vi "InitDC.vi"(8 "error in (no error)":errorcluster, 9 "_addr":u8, 10 "Motornum":u8, 11 "DCMotor in":refnum<class "DCMotor.lvclass">) -> (0 "error out":errorcluster, 3 "DCMotor out":refnum<class "DCMotor.lvclass">)   [LabVIEW 2022 SP3, in "Motorshield.lvlib" / "DCMotor.lvclass"]
uses:
  DCMotor.lvclass
  DCMotor.lvclass/DCMotor.ctl
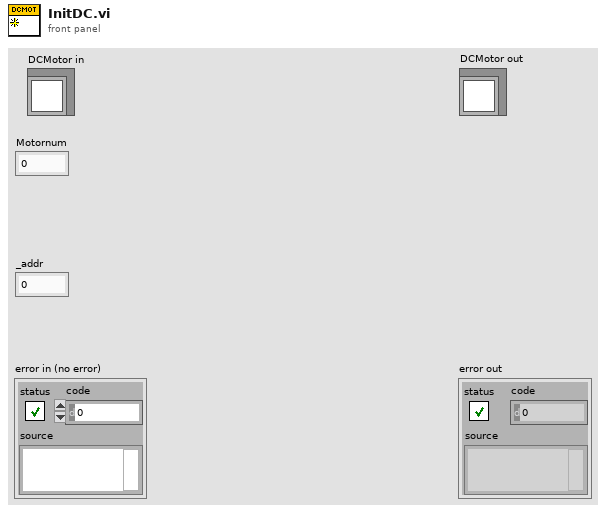
[diagram p1: front panel]
types:
  T1 = typedef "Motorshield.lvlib/DCMotor.lvclass/MotorInfo.ctl" = cluster{"PWMin":u8, "In1pin":u8, "In2pin":u8}
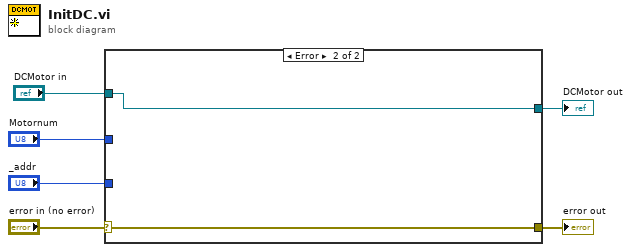
[diagram p0: block diagram]
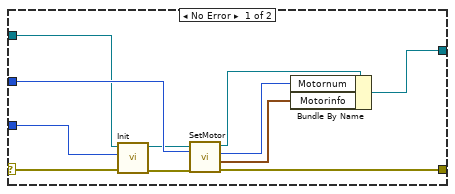
[diagram p2: hidden frame]
diagram:
  n1 = case shown="Error" "error in (no error)" {
    selector: "error in (no error)" -> [w11 w19]
    tunnel: [w16 w19] -> w5
    tunnel: [w17 w18] -> w4
    tunnel: "Motornum" -> [w12 _]
    tunnel: "_addr" -> [w8 _]
    tunnel: "DCMotor in" -> [w7 w18]
    frame No Error {
      n2 = call-dynamic "Init.vi"("error in (no error)"=w11, "_addr"=w8, "Motorshield in"=w7) -> ("error out"=w10:errorcluster, "Motorshield out"=w9:refnum<class "DCMotor.lvclass">)  [unwired: 7 in]
      n3 = call-dynamic "SetMotor.vi"("error in (no error)"=w10, "index(0..3)"=w12, "Motorshield in"=w9) -> ("error out"=w16:errorcluster, "Motorinfo"=w14:T1, "index"=w13:i32, "Motorshield out"=w15:refnum<class "DCMotor.lvclass">)  [unwired: 5 in]
      n4 = Bundle By Name(cluster=w15, "Motornum"=w13, "Motorinfo"=w14) -> (w17:refnum<class "DCMotor.lvclass">)
    }
    frame Error {
    }
  }
  "error out" <- w5
  "DCMotor out" <- w4
